vi "SS_DeviceStrip.vi"(6 "Main Cluster IN":T1, 8 "Error In":errorcluster, 9 "INI File Path":path, 11 "Info In":string="\nWaiting for TimerScope Trigger\n- IN: SS TimerScope Trigger\n- OUT: SET SS ThermoRec Received Trigger\nPulse Number is 231123\nPulse Type is 4\n\nDuration (s) is  2.000000\nDelay (s)  is  1.000000\nScan Period (ms) is  15\nNumber of Samples is  134\n\nDelay Started\nDelay Complete\nExternal Measurement of Delay (s): 1.000000\nACQUIRING DATA") -> (0 "Error Out":errorcluster, 3 "Info Out":string="\nWaiting for TimerScope Trigger\n- IN: SS TimerScope Trigger\n- OUT: SET SS ThermoRec Received Trigger\nPulse Number is 231123\nPulse Type is 4\n\nDuration (s) is  2.000000\nDelay (s)  is  1.000000\nScan Period (ms) is  15\nNumber of Samples is  134\n\nDelay Started\nDelay Complete\nExternal Measurement of Delay (s): 1.000000\nACQUIRING DATA", 4 "Main Cluster OUT":T1)   [LabVIEW 2016]
uses:
  Control/Control_Main.ctl
  Control/Control_ModuleArray.ctl
  <vilib>/Utility/file.llb/Read Delimited Spreadsheet (string).vi
panel:
  in  "Tab Control":enum32{"IN", "OUT", "SubVI Info"}(tab)
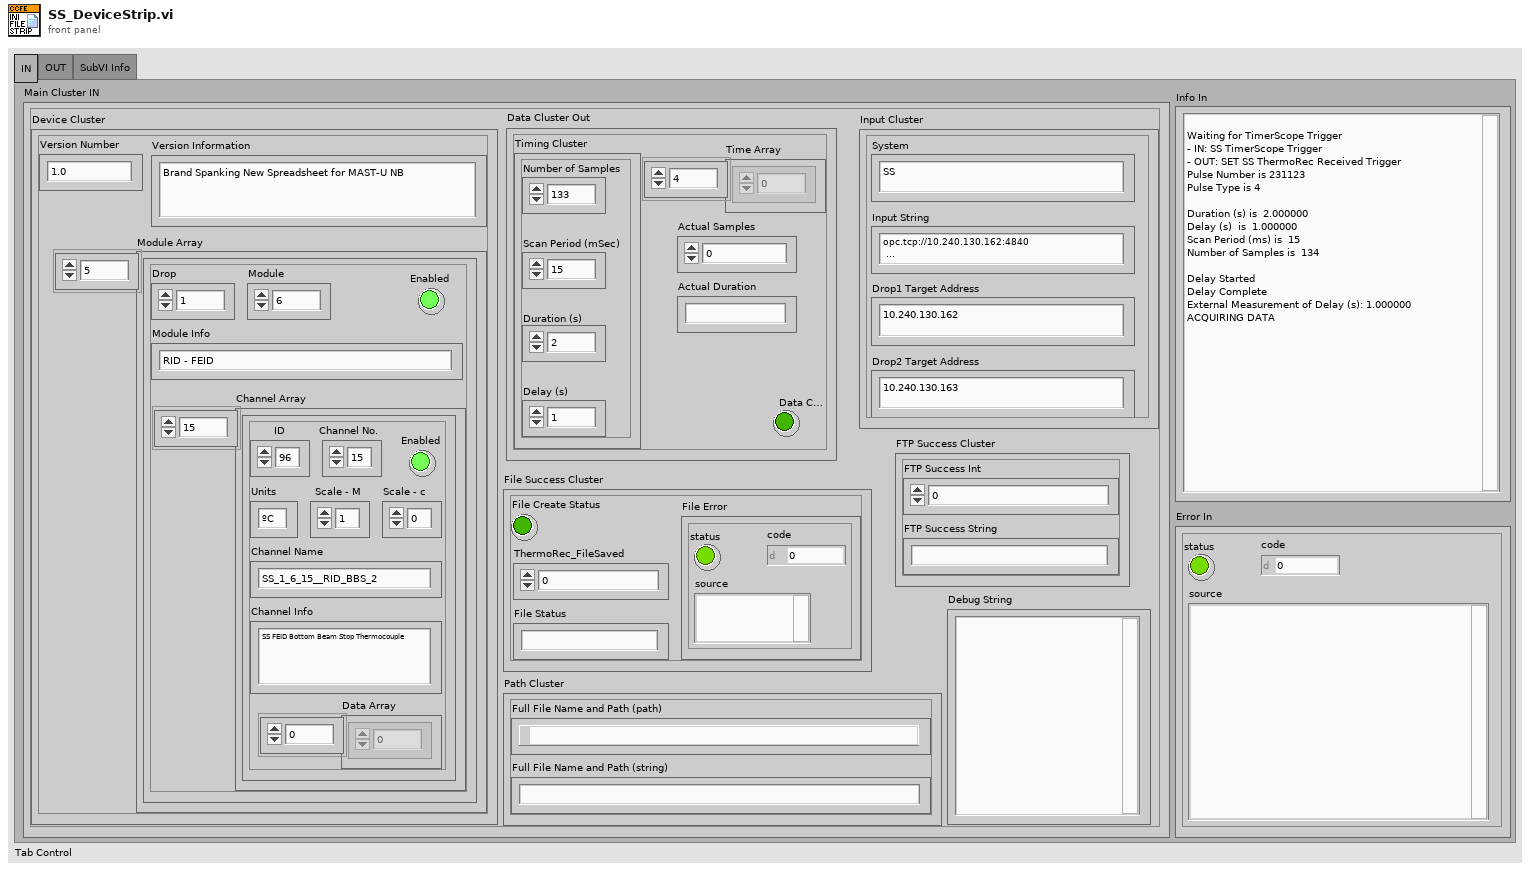
[diagram p1: front panel]
types:
  T1 = typedef "Control_Main.ctl" = cluster{"Device Cluster":cluster{"Module Array":T2, "Version Number":string, "Version Information":string}, "Input Cluster":cluster{"Input String":string, "Drop1 Target Address":string, "Drop2 Target Address":string, "System":string}, "Data Cluster Out":cluster{"Timing Cluster":cluster{"Number of Samples":i32, "Scan Period (mSec)":u32, "Duration (s)":dbl, "Delay (s)":dbl}, "Time Array":dbl[], "Actual Samples":i32, "Actual Duration":string, "Data Collection Error":bool}, "Path Cluster":cluster{"Full File Name and Path (path)":path, "Full File Name and Path (string)":string}, "File Success Cluster":cluster{"ThermoRec_FileSaved":i32, "File Create Status":bool, "File Error":errorcluster, "File Status":string}, "FTP Success Cluster":cluster{"FTP Success Int":i32, "FTP Success String":string}, "Debug String":string}
  T2 = typedef "Control_ModuleArray.ctl" = cluster{"Drop":i32, "Module":i32, "Module Info":string, "Enabled":bool, "Channel Array":cluster{"ID":i32, "Channel No.":i32, "Enabled":bool, "Channel Name":string, "Channel Info":string, "Units":string, "Scale - M":dbl, "Scale - c":dbl, "Data Array":dbl[]}[]}[]
  T3 = cluster{"Module Array":T2, "Version Number":string, "Version Information":string}
  T4 = cluster{"Drop":i32, "Module":i32, "Module Info":string, "Enabled":bool, "Channel Array":cluster{"ID":i32, "Channel No.":i32, "Enabled":bool, "Channel Name":string, "Channel Info":string, "Units":string, "Scale - M":dbl, "Scale - c":dbl, "Data Array":dbl[]}[]}
  T5 = cluster{"ID":i32, "Channel No.":i32, "Enabled":bool, "Channel Name":string, "Channel Info":string, "Units":string, "Scale - M":dbl, "Scale - c":dbl, "Data Array":dbl[]}[]
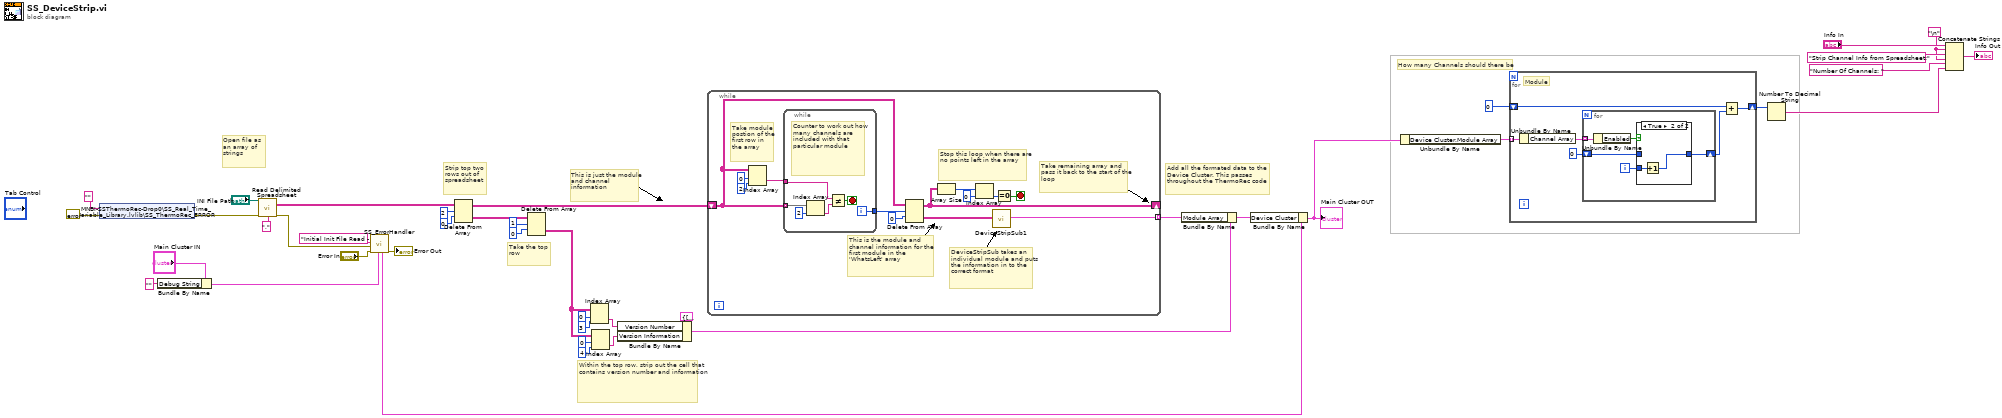
[diagram p0: block diagram]
diagram:
  w4 = "\n"
  # "Open file as an array of strings"
  # "How many Channels should there be"
  # "Add all the formated data to the Device Cluster. This passes throughout the ThermoRec code"
  # "This is just the module and channel information"
  # "Within the top row, strip out the cell that contains version number and information"
  # "Take the top row"
  # "Strip top two rows out of spreadsheet"
  n1 = shared-variable "MNBI-SSThermoRec-Drop0\\SS_Real_Time_Variable_Library.lvlib\\SS_ThermoRec_ERROR"("" ("SS_ThermoRec_ERROR"), error in=errorcluster {"status"=FALSE, "code"=0, "source"=""}) -> (error out=w20:errorcluster)
  n2 = Bundle By Name(cluster="Main Cluster IN", "Debug String"="") -> (w11:T1)
  n3 = call-poly <vilib>:"Read Delimited Spreadsheet.vi"("file path (dialog if empty)"="INI File Path", "error in (no error)"=w20, "delimiter (\\t)"=",") -> ("all rows"=w40:string[][], "error out"=w15:errorcluster)  [unwired: 7 in, 4 out]
  n4 = call "SS_ErrorHandler.vi"("Main Cluster IN"=w11, "Error In"="Error In", "SubVI Error"=w15, "SubVI Name"="Initial Init File Read - ") -> ("Error Out"=→"Error Out":errorcluster, "Main Cluster OUT"=w14:T1)  [unwired: 5 in, 1 out]
  n5 = Delete From Array(array=w40, length=2, index (row)=0) -> (deleted portion=w35:string[][], array with subset deleted=w26:string[][])  [unwired: 1 in]
  n6 = Delete From Array(array=w35, length=1, index (row)=0) -> (deleted portion=w29:string[][])  [unwired: 1 in, 1 out]
  n7 = Index Array(array=w29, index (row)=0, index (col)=3 ("disabled index (col)")) -> (element=w32:string)
  n8 = Index Array(array=w29, index (row)=0, index (col)=4 ("disabled index (col)")) -> (element=w28:string)
  n9 = Bundle By Name(cluster=T3 {"Module Array"=[], "Version Number"="", "Version Information"=""} ("Device Cluster"), "Version Number"=w32, "Version Information"=w28) -> (w27:T3)
  n10 = while {
    shift-right: [w49] -> _
    shift-left: w26 -> [w45]
    tunnel: [w42] -> w25 mode=indexing
    stop <- w47 stop-if-true
    # "Take remaining array and pass it back to the start of the loop"
    # "Stop this loop when there are no points left in the array"
    # "DeviceStripSub takes an individual module and puts the information in to the correct format"
    # "This is the module and channel information for the first module in the 'WhatsLeft' array"
    # "Take module postion of the first row in the array"
    n11 = Index Array(array=w45, index (row)=0 ("index"), index (col)=2 ("index")) -> (element=w43:string)
    n12 = while {
      tunnel: w45 -> [w60] mode=indexing
      tunnel: [w59] -> w54
      tunnel: w43 -> [w56]
      i -> [w59]
      stop <- w58 stop-if-true
      # "Counter to work out how many channels are included with that particular module"
      n13 = Index Array(array=w60, index=2) -> (element=w55:string)
      n14 = Not Equal?(x=w56, y=w55) -> (x != y?=w58:bool)
    }
    n15 = Delete From Array(array=w45, length=w54, index (row)=0) -> (deleted portion=w52:string[][], array with subset deleted=w49:string[][])  [unwired: 1 in]
    n16 = Array Size(array=w49) -> (size(s)=w50:i32[])
    n17 = Index Array(array=w50, index=0) -> (element=w48:i32)
    n18 = call "DeviceStripSub1.vi"("Individual Module Information Array"=w52) -> ("Formatted Module Information"=w42:T4)  [unwired: 10 in]
    n19 = Equal To 0?(x=w48) -> (x = 0?=w47:bool)
  }
  n20 = Bundle By Name(cluster=w27, "Module Array"=w25) -> (w23:T3)
  n21 = Bundle By Name(cluster=w14, "Device Cluster"=w23) -> (w7:T1)
  "Main Cluster OUT" <- w7
  n22 = Unbundle By Name(w7) -> ("Device Cluster.Module Array"=w10:T2)
  n23 = for {
    tunnel: w10 -> [w66] mode=indexing
    shift-right: [w61] -> w8
    shift-left: 0 -> [w63]
    # "Module"
    n24 = Unbundle By Name(w66) -> ("Channel Array"=w65:T5)
    n25 = for {
      tunnel: w65 -> [w71] mode=indexing
      shift-right: [w68] -> w62
      shift-left: 0 -> [w69]
      i -> [w67]
      n26 = Unbundle By Name(w71) -> ("Enabled"=w70:bool)
      n27 = case shown="True" w70 {
        tunnel: w69 -> [w72 _]
        tunnel: [w72 w73] -> w68
        tunnel: w67 -> [_ w74]
        frame False {
        }
        frame True {
          n28 = Increment(x=w74) -> (x+1=w73:i32)
        }
      }
    }
    n29 = Add(x=w63, y=w62) -> (x+y=w61:i32)
  }
  n30 = Number To Decimal String(number=w8) -> (decimal integer string=w2:string)  [unwired: 1 in]
  n31 = Concatenate Strings("Info In", w4, "Strip Channel Info from Spreadsheet:", w4, "Number Of Channels: ", w2) -> (→"Info Out":string)
